vi "main.vi"() -> ()   [LabVIEW 2018]
panel:
  out "1#NG":bool
  out "外观NG":bool
  in  "选项卡控件":enum32{"外观检测", "左出风口"}(tab)
  out "1#海绵":bool
  out "3#小齿":bool
  out "3#海绵":bool
  out "3#缓冲块":bool
  out "3#内叶片":bool
  out "3#卡扣4":bool
  out "3#卡扣3":bool
  out "3#卡扣2":bool
  out "3#卡扣1":bool
  out "3#外观4":bool
  out "3#外观3":bool
  out "3#外观2":bool
  out "3#外观1":bool
  out "2#小齿":bool
  out "2#海绵":bool
  out "2#缓冲块":bool
  out "2#内叶片":bool
  out "2#卡扣4":bool
  out "2#卡扣3":bool
  out "2#卡扣2":bool
  out "2#卡扣1":bool
  out "2#外观4":bool
  out "2#外观3":bool
  out "2#外观2":bool
  out "2#外观1":bool
  out "1#小齿":bool
  out "1#缓冲块":bool
  out "1#内叶片":bool
  out "1#卡扣4":bool
  out "1#卡扣3":bool
  out "1#卡扣2":bool
  out "1#卡扣1":bool
  out "1#外观4":bool
  out "1#外观3":bool
  out "1#外观2":bool
  out "1#外观1":bool
  in  "外观检测结果":string
  out "图片1":picture
  out "图片4":picture
  out "图片3":picture
  out "图片2":picture
  out "1#F拨钮右左锁":string
  out "1#F拨钮右左":string
  out "1#F拨钮左右锁":string
  out "1#F拨钮左右":string
  out "1#拨钮左右标准":string
  out "1#拨钮左右锁止标准":string
  out "1#拨钮右左标准":string
  out "1#拨钮右左锁止标准":string
  out "1#泄漏量结果":string
  out "1#压力结果":string
  out "1#泄漏量标准":string
  in  "1#F选项卡控件":enum32{"拨钮左->右", "拨钮右->左", "拨钮下->上", "拨钮上->下"}(tab)
  out "1#拨钮左右":T1(graph) caption="拨钮左右"
  out "1#拨钮右左":T1(graph) caption="拨钮右左"
  out "1#拨钮下上":T2(graph) caption="拨钮下上"
  out "1#拨钮上下":T2(graph) caption="拨钮上下"
  out "1#压力标准":string
  out "1#拨钮下上标准":string
  out "1#拨钮上下标准":string
  out "1#F拨钮上下":string
  out "1#F拨钮下上":string
  out "产品名称":string="请选择出风口型号..."
  in  "产品选择":enum32{"未选择", "1", "2"}(radio)=enum."1"
  out "ROBOT通讯状态":bool
  out "PLC通讯":bool
  out "时刻":string
  in  "参数":bool
  in  "退出":bool
  out "OK-NG":string
  # "泄漏检测"
  # "拨钮操作力（N）"
  # "项目"
  # "标准"
  # "结果"
  # "操作方向"
  # "力类型"
  # "标准"
  # "结果"
  # "滑动力"
  # "上->下"
  # "压力"
  # "滑动力"
  # "下->上"
  # "泄漏量"
  # "拨钮操作力（N）"
  # "操作方向"
  # "力类型"
  # "标准"
  # "结果"
  # "滑动力"
  # "左->右"
  # "锁止力"
  # "滑动力"
  # "右->左"
  # "锁止力"
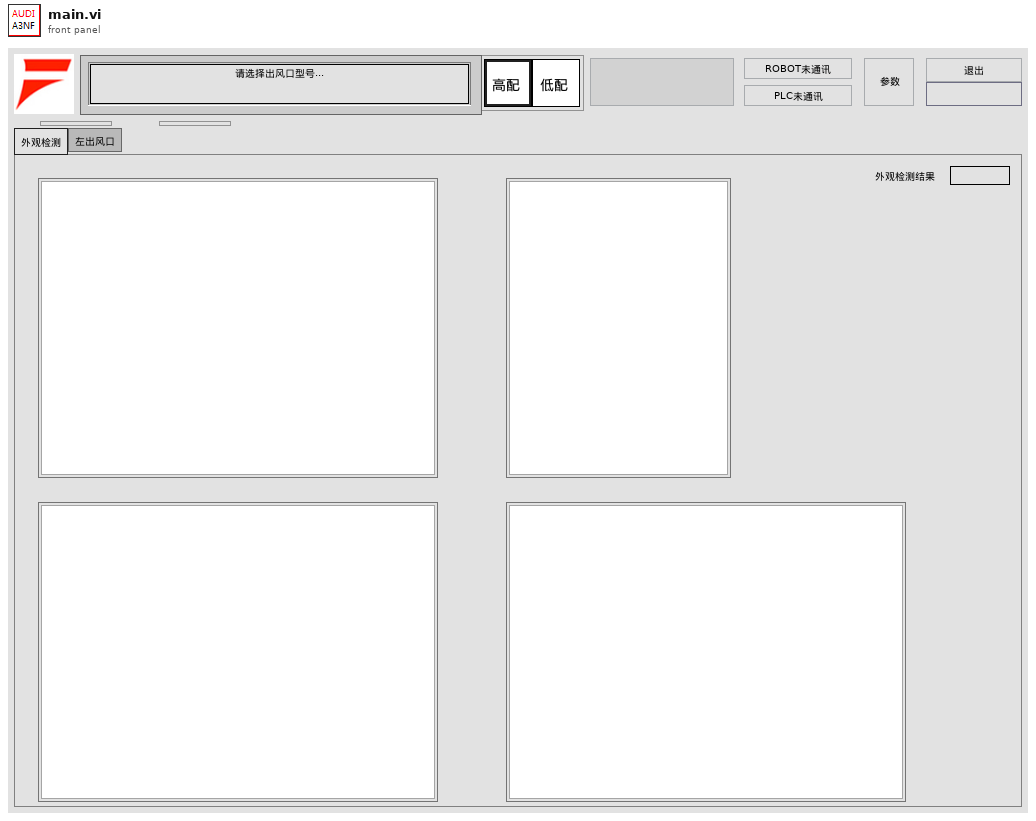
[diagram p1: front panel]
types:
  T1 = cluster{"力":sgl, "上限":sgl, "下限":sgl, "上参考":sgl, "下参考":sgl, "下参考 2":sgl}
  T2 = cluster{"力":sgl, "上限":sgl, "下限":sgl, "上参考":sgl, "下参考":sgl, "基准":sgl}
  T3 = enum8{"Enabled", "Disabled", "Disabled and Grayed Out"}
  T4 = cluster{"力":sgl, "上限":sgl, "下限":sgl, "上参考":sgl, "下参考":sgl, "下参考 2":sgl}[]
  T5 = enum32{"Invalid", "Standard", "Closed", "Hidden", "Minimized", "Maximized"}
  T6 = cluster{"压力":string, "泄漏量":string, "风门打开":string, "风门关闭":string, "LED电压":string, "LED电流":string, "拨钮左右":string, "拨钮左右锁止":string, "拨钮右左":string, "拨钮右左锁止":string, "拨钮上下":string, "拨钮下上":string, "轮盘关开":string, "轮盘关开锁止":string, "轮盘开关":string, "轮盘开关锁止":string}
  T7 = enum16{"Always On", "Always Off", "Off While Running"}
  T8 = cluster{"PLC就绪":bool, "ROBOT就绪":bool, "空动作":bool, "检测NG":bool, "检测结束":bool, "检测开始":bool, "初始化脉冲":bool, "1#检测NG":bool, "2#检测NG":bool, "3#检测NG":bool}
  T9 = cluster{"选择":enum16{"Fx", "Fy", "Fz", "Mx", "My", "Mz"}, "系数x":sgl, "系数+":sgl, "上限":sgl, "下限":sgl, "Ymax":dbl, "Ymin":dbl, "点数":dbl, "锁系数x":sgl, "锁上限":sgl, "锁下限":sgl, "锁系数+":sgl, "起点":dbl, "终点":dbl, "锁起点":dbl, "锁终点":dbl, "上参考":sgl, "下参考":sgl, "基准":sgl}
  T10 = cluster{"1#当前泄漏量":sgl, "1#稳定泄漏量":sgl, "1#当前压力":sgl, "1#稳定压力":sgl, "1#风门闭电压":sgl, "1#风门开电压":sgl, "1#LED电流":sgl, "1#LED电压":sgl, "2#当前泄漏量":sgl, "2#稳定泄漏量":sgl, "2#当前压力":sgl, "2#稳定压力":sgl, "2#风门闭电压":sgl, "2#风门开电压":sgl, "2#LED电流":sgl, "2#LED电压":sgl, "3#当前泄漏量":sgl, "3#稳定泄漏量":sgl, "3#当前压力":sgl, "3#稳定压力":sgl, "3#风门闭电压":sgl, "3#风门开电压":sgl, "3#LED电流":sgl, "3#LED电压":sgl}
  T11 = cluster{"泄漏量":bool, "风门开闭电检":bool, "LED电检":bool, "外观检测":bool, "1#轮盘关开":bool, "1#轮盘关开锁":bool, "1#轮盘开关":bool, "1#轮盘开关锁":bool, "1#拨钮左右":bool, "1#拨钮右左":bool, "1#拨钮上下":bool, "1#拨钮下上":bool, "2#轮盘关开":bool, "2#轮盘关开锁":bool, "2#轮盘开关":bool, "2#轮盘开关锁":bool, "2#拨钮左右":bool, "2#拨钮右左":bool, "2#拨钮上下":bool, "2#拨钮下上":bool, "3#轮盘关开":bool, "3#轮盘关开锁":bool, "3#轮盘开关":bool, "3#轮盘开关锁":bool, "3#拨钮左右":bool, "3#拨钮右左":bool, "3#拨钮上下":bool, "3#拨钮下上":bool}
  T12 = cluster{"1#泄漏量":bool, "1#风门闭电压":bool, "1#风门开电压":bool, "1#LED电压":bool, "1#LED电流":bool, "外观结果":bool, "2#泄漏量":bool, "2#风门闭电压":bool, "2#风门开电压":bool, "2#LED电压":bool, "2#LED电流":bool, "3#泄漏量":bool, "3#风门闭电压":bool, "3#风门开电压":bool, "3#LED电压":bool, "3#LED电流":bool}
  T13 = cluster{"主站IP":u32, "组号":u8, "帧号":u16, "时间戳":u64}
  T14 = cluster{"力":sgl, "上限":sgl, "下限":sgl, "上参考":sgl, "下参考":sgl, "基准":sgl}[]
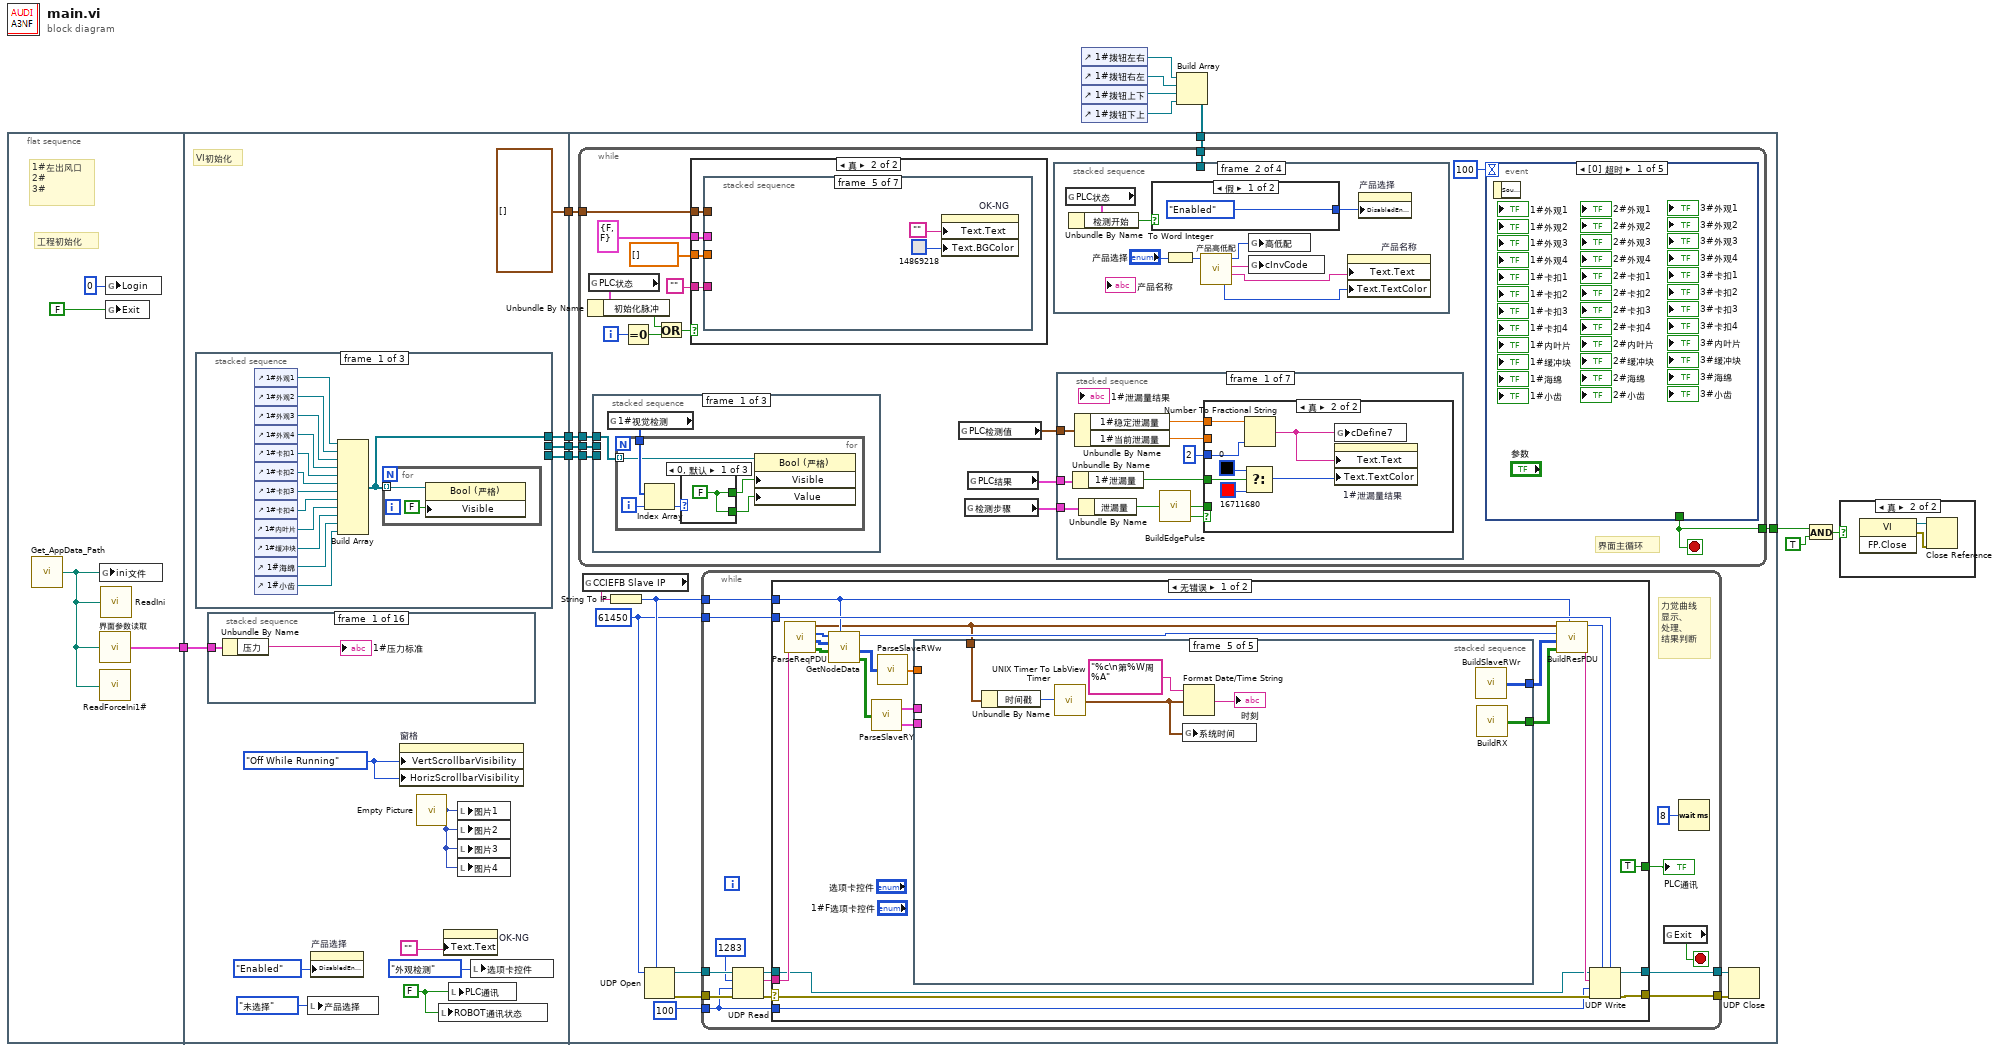
[diagram p0: block diagram]
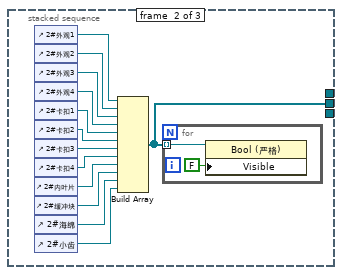
[diagram p2: hidden frame]
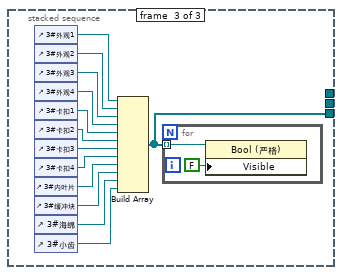
[diagram p3: hidden frame]
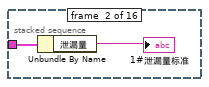
[diagram p4: hidden frame]
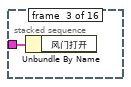
[diagram p5: hidden frame]
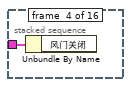
[diagram p6: hidden frame]
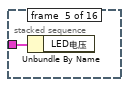
[diagram p7: hidden frame]
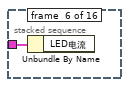
[diagram p8: hidden frame]
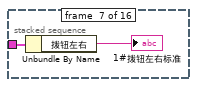
[diagram p9: hidden frame]
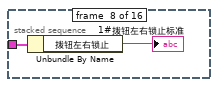
[diagram p10: hidden frame]
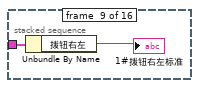
[diagram p11: hidden frame]
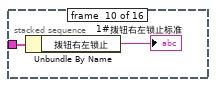
[diagram p12: hidden frame]
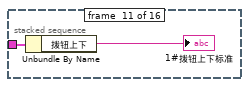
[diagram p13: hidden frame]
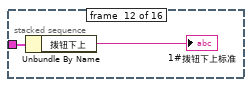
[diagram p14: hidden frame]
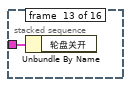
[diagram p15: hidden frame]
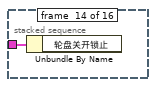
[diagram p16: hidden frame]
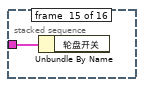
[diagram p17: hidden frame]
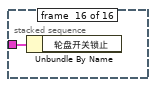
[diagram p18: hidden frame]
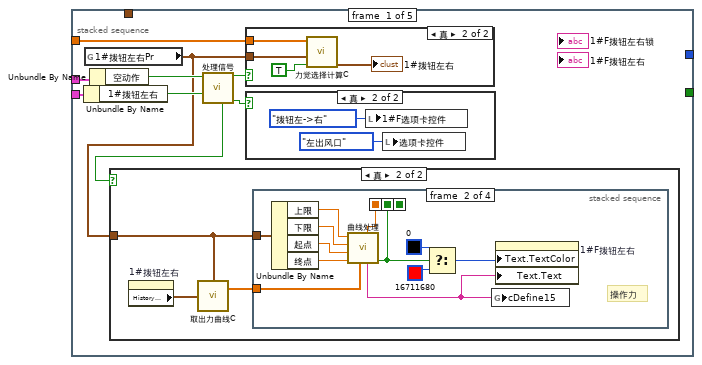
[diagram p19: hidden frame]
diagram:
  n1 = flat-sequence {
    tunnel: [w16] -> w9
    tunnel: [w29] -> w10
    tunnel: w9 -> [w26]
    tunnel: [w24] -> w8
    tunnel: [w23] -> w7
    tunnel: [T4 [] ("历史数据")] -> w6
    tunnel: [w112] -> w12
    tunnel: w10 -> [w105]
    tunnel: w8 -> [w102]
    tunnel: w7 -> [w101]
    tunnel: w6 -> [w100]
    tunnel: w1 -> [w99]
    frame #0 {
      # "1#左出风口\n2#\n3#"
      # "工程初始化"
      n2 = call "Get_AppData_Path.vi"() -> ("path"=w15:path)  [unwired: 1 in]
      n3 = global write "全局 1.vi" "ini文件"(w15) -> ()
      n4 = call "界面参数读取.vi"("路径"=w15) -> ("标准"=w16:T6)
      n5 = call "ReadForceIni1#.vi"("configuration file path"=w15) -> ()  [unwired: 1 in]
      n6 = call "ReadIni.vi"("configuration file path"=w15) -> ()  [unwired: 1 in]
      n7 = global write "全局 1.vi" "Login"(0 ("Login")) -> ()
      n8 = global write "全局 1.vi" "Exit"(FALSE ("退出")) -> ()
    }
    frame #1 {
      w25 = T7."Off While Running" ("垂直滚动条可见")
      w27 = FALSE
      # "VI初始化"
      n9 = stacked-sequence {
        tunnel: [w42 _ _] -> w29
        tunnel: [_ w45 _] -> w24
        tunnel: [_ _ w60] -> w23
        frame #0 {
          n10 = control-ref of="1#外观1"() -> (w30:refnum<vi>)
          n11 = control-ref of="1#外观2"() -> (w31:refnum<vi>)
          n12 = control-ref of="1#外观3"() -> (w32:refnum<vi>)
          n13 = control-ref of="1#外观4"() -> (w33:refnum<vi>)
          n14 = control-ref of="1#卡扣1"() -> (w34:refnum<vi>)
          n15 = control-ref of="1#卡扣2"() -> (w41:refnum<vi>)
          n16 = control-ref of="1#卡扣3"() -> (w40:refnum<vi>)
          n17 = control-ref of="1#卡扣4"() -> (w39:refnum<vi>)
          n18 = control-ref of="1#内叶片"() -> (w38:refnum<vi>)
          n19 = control-ref of="1#缓冲块"() -> (w37:refnum<vi>)
          n20 = control-ref of="1#海绵"() -> (w36:refnum<vi>)
          n21 = control-ref of="1#小齿"() -> (w35:refnum<vi>)
          n22 = Build Array(w30, w31, w32, w33, w34, w41, w40, w39, w38, w37, w36, w35) -> (w42:refnum<vi>[])
          n23 = for {
            tunnel: w42 -> [w43] mode=indexing
            n24 = property class="Bool (严格)"(reference=w43, "Visible"=FALSE ("可见")) -> ()  [unwired: 1 in, 2 out]
          }
        }
        frame #1 {
          n25 = control-ref of="2#外观1"() -> (w46:refnum<vi>)
          n26 = control-ref of="2#外观2"() -> (w47:refnum<vi>)
          n27 = control-ref of="2#外观3"() -> (w48:refnum<vi>)
          n28 = control-ref of="2#外观4"() -> (w49:refnum<vi>)
          n29 = control-ref of="2#卡扣1"() -> (w50:refnum<vi>)
          n30 = control-ref of="2#卡扣2"() -> (w57:refnum<vi>)
          n31 = control-ref of="2#卡扣3"() -> (w56:refnum<vi>)
          n32 = control-ref of="2#卡扣4"() -> (w55:refnum<vi>)
          n33 = control-ref of="2#内叶片"() -> (w54:refnum<vi>)
          n34 = control-ref of="2#缓冲块"() -> (w53:refnum<vi>)
          n35 = control-ref of="2#海绵"() -> (w52:refnum<vi>)
          n36 = control-ref of="2#小齿"() -> (w51:refnum<vi>)
          n37 = Build Array(w46, w47, w48, w49, w50, w57, w56, w55, w54, w53, w52, w51) -> (w45:refnum<vi>[])
          n38 = for {
            tunnel: w45 -> [w58] mode=indexing
            n39 = property class="Bool (严格)"(reference=w58, "Visible"=FALSE ("可见")) -> ()  [unwired: 1 in, 2 out]
          }
        }
        frame #2 {
          n40 = control-ref of="3#外观1"() -> (w61:refnum<vi>)
          n41 = control-ref of="3#外观2"() -> (w62:refnum<vi>)
          n42 = control-ref of="3#外观3"() -> (w63:refnum<vi>)
          n43 = control-ref of="3#外观4"() -> (w64:refnum<vi>)
          n44 = control-ref of="3#卡扣1"() -> (w65:refnum<vi>)
          n45 = control-ref of="3#卡扣2"() -> (w72:refnum<vi>)
          n46 = control-ref of="3#卡扣3"() -> (w71:refnum<vi>)
          n47 = control-ref of="3#卡扣4"() -> (w70:refnum<vi>)
          n48 = control-ref of="3#内叶片"() -> (w69:refnum<vi>)
          n49 = control-ref of="3#缓冲块"() -> (w68:refnum<vi>)
          n50 = control-ref of="3#海绵"() -> (w67:refnum<vi>)
          n51 = control-ref of="3#小齿"() -> (w66:refnum<vi>)
          n52 = Build Array(w61, w62, w63, w64, w65, w72, w71, w70, w69, w68, w67, w66) -> (w60:refnum<vi>[])
          n53 = for {
            tunnel: w60 -> [w73] mode=indexing
            n54 = property class="Bool (严格)"(reference=w73, "Visible"=FALSE ("可见")) -> ()  [unwired: 1 in, 2 out]
          }
        }
      }
      n55 = stacked-sequence {
        tunnel: w26 -> [w76 w78 w79 w80 w81 w82 w84 w86 w88 w90 w92 w94 w95 w96 w97 w98]
        frame #0 {
          n56 = Unbundle By Name(w76) -> ("压力"=→"1#压力标准":string)
        }
        frame #1 {
          n57 = Unbundle By Name(w78) -> ("泄漏量"=→"1#泄漏量标准":string)
        }
        frame #2 {
          n58 = Unbundle By Name(w79) -> ()  [unwired: 1 out]
        }
        frame #3 {
          n59 = Unbundle By Name(w80) -> ()  [unwired: 1 out]
        }
        frame #4 {
          n60 = Unbundle By Name(w81) -> ()  [unwired: 1 out]
        }
        frame #5 {
          n61 = Unbundle By Name(w82) -> ()  [unwired: 1 out]
        }
        frame #6 {
          n62 = Unbundle By Name(w84) -> ("拨钮左右"=→"1#拨钮左右标准":string)
        }
        frame #7 {
          n63 = Unbundle By Name(w86) -> ("拨钮左右锁止"=→"1#拨钮左右锁止标准":string)
        }
        frame #8 {
          n64 = Unbundle By Name(w88) -> ("拨钮右左"=→"1#拨钮右左标准":string)
        }
        frame #9 {
          n65 = Unbundle By Name(w90) -> ("拨钮右左锁止"=→"1#拨钮右左锁止标准":string)
        }
        frame #10 {
          n66 = Unbundle By Name(w92) -> ("拨钮上下"=→"1#拨钮上下标准":string)
        }
        frame #11 {
          n67 = Unbundle By Name(w94) -> ("拨钮下上"=→"1#拨钮下上标准":string)
        }
        frame #12 {
          n68 = Unbundle By Name(w95) -> ()  [unwired: 1 out]
        }
        frame #13 {
          n69 = Unbundle By Name(w96) -> ()  [unwired: 1 out]
        }
        frame #14 {
          n70 = Unbundle By Name(w97) -> ()  [unwired: 1 out]
        }
        frame #15 {
          n71 = Unbundle By Name(w98) -> ()  [unwired: 1 out]
        }
      }
      n72 = local write "产品选择"(enum32{"未选择", "1", "2"}."未选择" ("产品选择")) -> ()
      n73 = property on="产品选择" class="RadioBtnsControl (严格)"("DisabledEnum"=T3."Enabled" ("禁用")) -> ()  [unwired: 2 in, 2 out]
      n74 = property on="窗格" class="Pane"("VertScrollbarVisibility"=w25, "HorizScrollbarVisibility"=w25) -> ()  [unwired: 2 in, 2 out]
      n75 = call "Empty Picture"() -> ("empty picture"=w19:picture)
      n76 = local write "ROBOT通讯状态"(w27) -> ()
      n77 = property on="OK-NG" class="Str"("Text.Text"="") -> ()  [unwired: 2 in, 2 out]
      n78 = local write "PLC通讯"(w27) -> ()
      n79 = local write "图片1"(w19) -> ()
      n80 = local write "图片2"(w19) -> ()
      n81 = local write "图片3"(w19) -> ()
      n82 = local write "图片4"(w19) -> ()
      n83 = local write "选项卡控件"(enum32{"外观检测", "左出风口"}."外观检测" ("选项卡控件")) -> ()
    }
    frame #2 {
      w106 = u16 61450 ("端口")
      n84 = while {
        tunnel: [w362] -> w112
        tunnel: w105 -> [w361]
        tunnel: w102 -> [w354]
        tunnel: w101 -> [w353]
        tunnel: w100 -> [w347]
        tunnel: w99 -> [w346]
        i -> [w352]
        stop <- w362 stop-if-true
        # "界面主循环"
        n85 = global read "全局 1.vi" "PLC状态"() -> (w360:T8)
        n86 = Unbundle By Name(w360) -> ("初始化脉冲"=w350:bool)
        n87 = stacked-sequence {
          tunnel: w361 -> [w364 _ _]
          tunnel: w354 -> [_ w377 _]
          tunnel: w353 -> [_ _ w390]
          frame #0 {
            n88 = global read "全局 1.vi" "1#视觉检测"() -> (w365:u16[])
            n89 = for {
              tunnel: w364 -> [w366] mode=indexing
              tunnel: w365 -> [w371]
              i -> [w370]
              n90 = Index Array(array=w371, index=w370) -> (element=w369:u16)
              n91 = case shown="0, 默认" w369 {
                tunnel: [w372 TRUE TRUE] -> w368
                tunnel: [w372 FALSE TRUE] -> w367
                frame 0, Default {
                  w372 = FALSE
                }
                frame 1 {
                }
                frame 2 {
                }
              }
              n92 = property class="Bool (严格)"(reference=w366, "Visible"=w368, "Value"=w367) -> ()  [unwired: 1 in, 2 out]
            }
          }
          frame #1 {
            n93 = global read "全局 1.vi" "2#视觉检测"() -> (w378:u16[])
            n94 = for {
              tunnel: w377 -> [w379] mode=indexing
              tunnel: w378 -> [w384]
              i -> [w383]
              n95 = Index Array(array=w384, index=w383) -> (element=w382:u16)
              n96 = case shown="0, 默认" w382 {
                tunnel: [w385 TRUE TRUE] -> w381
                tunnel: [w385 FALSE TRUE] -> w380
                frame 0, Default {
                  w385 = FALSE
                }
                frame 1 {
                }
                frame 2 {
                }
              }
              n97 = property class="Bool (严格)"(reference=w379, "Visible"=w381, "Value"=w380) -> ()  [unwired: 1 in, 2 out]
            }
          }
          frame #2 {
            n98 = global read "全局 1.vi" "3#视觉检测"() -> (w391:u16[])
            n99 = for {
              tunnel: w390 -> [w392] mode=indexing
              tunnel: w391 -> [w397]
              i -> [w396]
              n100 = Index Array(array=w397, index=w396) -> (element=w395:u16)
              n101 = case shown="0, 默认" w395 {
                tunnel: [w398 TRUE TRUE] -> w394
                tunnel: [w398 FALSE TRUE] -> w393
                frame 0, Default {
                  w398 = FALSE
                }
                frame 1 {
                }
                frame 2 {
                }
              }
              n102 = property class="Bool (严格)"(reference=w392, "Visible"=w394, "Value"=w393) -> ()  [unwired: 1 in, 2 out]
            }
          }
        }
        n103 = Equal To 0?(x=w352) -> (x = 0?=w351:bool)
        n104 = Or(x=w350, y=w351) -> (x .or. y?=w349:bool)
        n105 = case shown="真" w349 {
          tunnel: cluster{bool, bool} {FALSE, FALSE} -> [_ w569]
          tunnel: sgl[] [] ("历史数据") -> [_ w568]
          tunnel: w347 -> [_ w567]
          tunnel: "" -> [_ w566]
          frame False {
          }
          frame True {
            n106 = stacked-sequence {
              tunnel: w569 -> [w578 w587 w596 w605 _ _ _]
              tunnel: w568 -> [_ _ _ _ _ _ _]
              tunnel: w567 -> [w570 w579 w589 w598 _ _ _]
              tunnel: w566 -> [w571 w580 w588 w597 _ w608 w610]
              frame #0 {
                n107 = global write "全局F结果.vi" "1#拨钮左右力检"(w578) -> ()
                n108 = global read "全局F参数.vi" "1#拨钮左右Pr"() -> (w576:T9)
                n109 = local write "1#F拨钮左右锁"(w571) -> ()
                n110 = local write "1#F拨钮左右"(w571) -> ()
                n111 = Unbundle By Name(w576) -> ("点数"=w577:dbl, "Ymax"=w573:dbl, "Ymin"=w572:dbl)
                n112 = Decrement(x=w577) -> (x-1=w575:dbl)
                n113 = property on="1#拨钮左右" class="WFChart (严格)"("History Data"=w570, "XScale.Minimum"=0.0, "XScale.Maximum"=w575, "YScale.Maximum"=w573, "YScale.Minimum"=w572) -> ()  [unwired: 2 in, 2 out]
              }
              frame #1 {
                n114 = global write "全局F结果.vi" "1#拨钮右左力检"(w587) -> ()
                n115 = global read "全局F参数.vi" "1#拨钮右左Pr"() -> (w586:T9)
                n116 = local write "1#F拨钮右左"(w580) -> ()
                n117 = local write "1#F拨钮右左锁"(w580) -> ()
                n118 = Unbundle By Name(w586) -> ("点数"=w585:dbl, "Ymax"=w584:dbl, "Ymin"=w583:dbl)
                n119 = Decrement(x=w585) -> (x-1=w582:dbl)
                n120 = property on="1#拨钮右左" class="WFChart (严格)"("History Data"=w579, "XScale.Minimum"=0.0 ("X标尺.范围:最大值"), "XScale.Maximum"=w582, "YScale.Maximum"=w584, "YScale.Minimum"=w583) -> ()  [unwired: 2 in, 2 out]
              }
              frame #2 {
                n121 = global read "全局F参数.vi" "1#拨钮下上Pr"() -> (w595:T9)
                n122 = global write "全局F结果.vi" "1#拨钮下上力检"(w596) -> ()
                n123 = local write "1#F拨钮下上"(w588) -> ()
                n124 = Unbundle By Name(w595) -> ("点数"=w594:dbl, "Ymax"=w591:dbl, "Ymin"=w590:dbl)
                n125 = Decrement(x=w594) -> (x-1=w593:dbl)
                n126 = property on="1#拨钮下上" class="WFChart (严格)"("History Data"=w589, "XScale.Minimum"=0.0 ("X标尺.范围:最大值"), "XScale.Maximum"=w593, "YScale.Maximum"=w591, "YScale.Minimum"=w590) -> ()  [unwired: 2 in, 2 out]
              }
              frame #3 {
                n127 = global write "全局F结果.vi" "1#拨钮上下力检"(w605) -> ()
                n128 = global read "全局F参数.vi" "1#拨钮上下Pr"() -> (w604:T9)
                n129 = local write "1#F拨钮上下"(w597) -> ()
                n130 = Unbundle By Name(w604) -> ("点数"=w603:dbl, "Ymax"=w600:dbl, "Ymin"=w599:dbl)
                n131 = Decrement(x=w603) -> (x-1=w602:dbl)
                n132 = property on="1#拨钮上下" class="WFChart (严格)"("History Data"=w598, "XScale.Minimum"=0.0 ("X标尺.范围:最大值"), "XScale.Maximum"=w602, "YScale.Maximum"=w600, "YScale.Minimum"=w599) -> ()  [unwired: 2 in, 2 out]
              }
              frame #4 {
                n133 = property on="OK-NG" class="Str"("Text.Text"="", "Text.BGColor"=u32 14869218) -> ()  [unwired: 2 in, 2 out]
              }
              frame #5 {
                n134 = local write "1#泄漏量结果"(w608) -> ()
                n135 = local write "1#压力结果"(w608) -> ()
              }
              frame #6 {
                w609 = FALSE
                n136 = local write "外观检测结果"(w610) -> ()
                n137 = local write "外观NG"(w609) -> ()
                n138 = local write "1#NG"(w609) -> ()
              }
            }
          }
        }
        n139 = global read "全局 1.vi" "PLC检测值"() -> (w358:T10)
        n140 = global read "全局 1.vi" "检测步骤"() -> (w359:T11)
        n141 = global read "全局 1.vi" "PLC结果"() -> (w357:T12)
        n142 = stacked-sequence {
          tunnel: w346 -> [_ _ _ w557]
          frame #0 {
            n143 = global read "全局 1.vi" "PLC状态"() -> (w531:T8)
            n144 = global read "全局 1.vi" "PC状态"() -> (w530:cluster{"PLC就绪":bool, "空动作中":bool})
            n145 = Bundle By Name(cluster=w530, "PLC就绪"=TRUE) -> (w528:cluster{"PLC就绪":bool, "空动作中":bool})
            n146 = Unbundle By Name(w531) -> ("ROBOT就绪"=→"ROBOT通讯状态":bool, "1#检测NG"=→"1#NG":bool)
            n147 = global write "全局 1.vi" "PC状态"(w528) -> ()
          }
          frame #1 {
            n148 = global read "全局 1.vi" "PLC状态"() -> (w541:T8)
            n149 = Unbundle By Name(w541) -> ("检测开始"=w540:bool)
            n150 = case shown="假" w540 {
              tunnel: [T3."Enabled" ("禁用") T3."Disabled and Grayed Out" ("禁用")] -> w539
              frame False {
              }
              frame True {
              }
            }
            n151 = To Word Integer(number="产品选择") -> (16bit integer=w537:i16)
            n152 = call "产品高低配.vi"("选择"=w537) -> ("颜色"=w534:u32, "产品名称"=w533:string, "物料编号"=w535:string, "高低配"=w536:i16)  [unwired: 5 in]
            n153 = global write "全局 1.vi" "高低配"(w536) -> ()
            n154 = global write "全局SQL.vi" "cInvCode"(w535) -> ()
            n155 = property on="产品名称" class="Str"("Text.Text"=w533, "Text.TextColor"=w534) -> ()  [unwired: 2 in, 2 out]
            n156 = property on="产品选择" class="RadioBtnsControl (严格)"("DisabledEnum"=w539) -> ()  [unwired: 2 in, 2 out]
          }
          frame #2 {
            n157 = global read "全局 1.vi" "PLC状态"() -> (w546:T8)
            n158 = Unbundle By Name(w546) -> ("检测NG"=w544:bool, "检测结束"=w545:bool)
            n159 = case shown="真" w545 {
              tunnel: w544 -> [_ w547]
              frame False {
              }
              frame True {
                n160 = case shown="假" w547 {
                  tunnel: ["合格" "不合格"] -> w550
                  tunnel: [u32 6618880 u32 16711680] -> w549
                  tunnel: [u32 0 u32 16448250] -> w548
                  frame False {
                  }
                  frame True {
                  }
                }
                n161 = property on="OK-NG" class="Str"("Text.Text"=w550, "Text.BGColor"=w549, "Text.TextColor"=w548) -> ()  [unwired: 2 in, 2 out]
              }
            }
          }
          frame #3 {
            n162 = global read "全局 1.vi" "PLC状态"() -> (w563:T8)
            n163 = Unbundle By Name(w563) -> ("检测NG"=w558:bool, "检测结束"=w559:bool)
            n164 = Compound Arithmetic op=AND ("复合运算")(w559, FALSE ("值")) -> (w562:bool)
            n165 = call "BuildEdgePulse.vi"("输入"=w562) -> ("下降沿"=w560:bool)  [unwired: 2 in, 2 out]
            n166 = case shown="真" w560 {
              tunnel: w558 -> [_ w565]
              tunnel: w557 -> [_ w564]
              frame False {
              }
              frame True {
                n167 = call "WriteDB.vi"("NG?"=w565, "曲线数组"=w564) -> ()  [unwired: 3 in]
              }
            }
          }
        }
        n168 = stacked-sequence {
          tunnel: w359 -> [w412 w436 w459 w474 w489 w503 w514]
          tunnel: w358 -> [w409 w433 w456 w471 w486 w500 _]
          tunnel: w357 -> [w405 w429 w453 w468 w483 w497 w511]
          frame #0 {
            n169 = Unbundle By Name(w405) -> ("1#泄漏量"=w404:bool)
            n170 = Unbundle By Name(w409) -> ("1#稳定泄漏量"=w407:sgl, "1#当前泄漏量"=w408:sgl)
            n171 = Unbundle By Name(w412) -> ("泄漏量"=w411:bool)
            n172 = call "BuildEdgePulse.vi"("输入"=w411) -> ("下降沿"=w410:bool, "输出"=w406:bool)  [unwired: 2 in, 1 out]
            n173 = case shown="真" w410 {
              tunnel: w408 -> [w415 _]
              tunnel: w407 -> [_ w426]
              tunnel: w406 -> [w414 _]
              tunnel: w404 -> [_ w425]
              tunnel: i16 2 ("精度(6)") -> [w413 w422]
              frame False {
                n174 = case shown="真" w414 {
                  tunnel: w415 -> [_ w419]
                  tunnel: w413 -> [_ w418]
                  frame False {
                  }
                  frame True {
                    n175 = Number To Fractional String(number=w419, precision (6)=w418) -> (F-format string=w416:string)  [unwired: 2 in]
                    n176 = property on="1#泄漏量结果" class="Str"("Text.Text"=w416, "Text.TextColor"=u32 0) -> ()  [unwired: 2 in, 2 out]
                  }
                }
              }
              frame True {
                n177 = Select(t=u32 0, s=w425, f=u32 16711680) -> (s? t:f=w421:u32)
                n178 = Number To Fractional String(number=w426, precision (6)=w422) -> (F-format string=w420:string)  [unwired: 2 in]
                n179 = global write "全局SQL.vi" "cDefine7"(w420) -> ()
                n180 = property on="1#泄漏量结果" class="Str"("Text.Text"=w420, "Text.TextColor"=w421) -> ()  [unwired: 2 in, 2 out]
              }
            }
          }
          frame #1 {
            n181 = Unbundle By Name(w429) -> ("1#泄漏量"=w428:bool)
            n182 = Unbundle By Name(w433) -> ("1#稳定压力"=w431:sgl, "1#当前压力"=w432:sgl)
            n183 = Unbundle By Name(w436) -> ("泄漏量"=w435:bool)
            n184 = call "BuildEdgePulse.vi"("输入"=w435) -> ("下降沿"=w434:bool, "输出"=w430:bool)  [unwired: 2 in, 1 out]
            n185 = case shown="假" w434 {
              tunnel: w432 -> [w439 _]
              tunnel: w431 -> [_ w449]
              tunnel: w430 -> [w438 _]
              tunnel: w428 -> [_ w448]
              tunnel: i16 1 ("精度(6)") -> [w437 w444]
              frame False {
                n186 = case shown="真" w438 {
                  tunnel: w439 -> [_ w441]
                  tunnel: w437 -> [_ w440]
                  frame False {
                  }
                  frame True {
                    n187 = Number To Fractional String(number=w441, precision (6)=w440) -> (F-format string=w443:string)  [unwired: 2 in]
                    n188 = property on="1#压力结果" class="Str"("Text.Text"=w443, "Text.TextColor"=u32 0) -> ()  [unwired: 2 in, 2 out]
                  }
                }
              }
              frame True {
                n189 = Select(t=u32 0, s=w448, f=u32 16711680) -> (s? t:f=w445:u32)
                n190 = Number To Fractional String(number=w449, precision (6)=w444) -> (F-format string=w450:string)  [unwired: 2 in]
                n191 = property on="1#压力结果" class="Str"("Text.Text"=w450, "Text.TextColor"=w445) -> ()  [unwired: 2 in, 2 out]
              }
            }
          }
          frame #2 {
            n192 = Unbundle By Name(w453) -> ("1#风门开电压"=w452:bool)
            n193 = Unbundle By Name(w459) -> ("风门开闭电检"=w458:bool)
            n194 = Unbundle By Name(w456) -> ("1#风门开电压"=w455:sgl)
            n195 = call "BuildEdgePulse.vi"("输入"=w458) -> ("下降沿"=w457:bool, "输出"=w454:bool)  [unwired: 2 in, 1 out]
            n196 = case shown="真" w457 {
              tunnel: w455 -> [_ w465]
              tunnel: w454 -> [_ _]
              tunnel: w452 -> [_ w464]
              tunnel: i16 2 ("精度(6)") -> [_ w461]
              frame False {
              }
              frame True {
                n197 = Number To Fractional String(number=w465, precision (6)=w461) -> (F-format string=w460:string)  [unwired: 2 in]
                n198 = Select(t=u32 0, s=w464, f=u32 16711680) -> ()  [unwired: 1 out]
                n199 = global write "全局SQL.vi" "cDefine17"(w460) -> ()
              }
            }
          }
          frame #3 {
            n200 = Unbundle By Name(w468) -> ("1#风门闭电压"=w467:bool)
            n201 = Unbundle By Name(w474) -> ("风门开闭电检"=w473:bool)
            n202 = Unbundle By Name(w471) -> ("1#风门闭电压"=w470:sgl)
            n203 = call "BuildEdgePulse.vi"("输入"=w473) -> ("下降沿"=w472:bool, "输出"=w469:bool)  [unwired: 2 in, 1 out]
            n204 = case shown="真" w472 {
              tunnel: w470 -> [_ w480]
              tunnel: w469 -> [_ _]
              tunnel: w467 -> [_ w479]
              tunnel: i16 2 ("精度(6)") -> [_ w476]
              frame False {
              }
              frame True {
                n205 = Number To Fractional String(number=w480, precision (6)=w476) -> (F-format string=w475:string)  [unwired: 2 in]
                n206 = Select(t=u32 0, s=w479, f=u32 16711680) -> ()  [unwired: 1 out]
                n207 = global write "全局SQL.vi" "cDefine18"(w475) -> ()
              }
            }
          }
          frame #4 {
            n208 = Unbundle By Name(w483) -> ("1#LED电压"=w482:bool)
            n209 = Unbundle By Name(w489) -> ("LED电检"=w488:bool)
            n210 = Unbundle By Name(w486) -> ("1#LED电压"=w485:sgl)
            n211 = call "BuildEdgePulse.vi"("输入"=w488) -> ("下降沿"=w487:bool, "输出"=w484:bool)  [unwired: 2 in, 1 out]
            n212 = case shown="真" w487 {
              tunnel: w485 -> [_ w494]
              tunnel: w484 -> [_ _]
              tunnel: w482 -> [_ w493]
              tunnel: i16 2 ("精度(6)") -> [_ w490]
              frame False {
              }
              frame True {
                n213 = Number To Fractional String(number=w494, precision (6)=w490) -> ()  [unwired: 2 in, 1 out]
                n214 = Select(t=u32 0, s=w493, f=u32 16711680) -> ()  [unwired: 1 out]
              }
            }
          }
          frame #5 {
            n215 = Unbundle By Name(w497) -> ("1#LED电流"=w496:bool)
            n216 = Unbundle By Name(w500) -> ("1#LED电流"=w499:sgl)
            n217 = Unbundle By Name(w503) -> ("LED电检"=w502:bool)
            n218 = call "BuildEdgePulse.vi"("输入"=w502) -> ("下降沿"=w501:bool, "输出"=w498:bool)  [unwired: 2 in, 1 out]
            n219 = case shown="真" w501 {
              tunnel: w499 -> [_ w509]
              tunnel: w498 -> [_ _]
              tunnel: w496 -> [_ w508]
              tunnel: i16 2 ("精度(6)") -> [_ w505]
              frame False {
              }
              frame True {
                n220 = Number To Fractional String(number=w509, precision (6)=w505) -> (F-format string=w504:string)  [unwired: 2 in]
                n221 = Select(t=u32 0, s=w508, f=u32 16711680) -> ()  [unwired: 1 out]
                n222 = global write "全局SQL.vi" "cDefine8"(w504) -> ()
              }
            }
          }
          frame #6 {
            n223 = Unbundle By Name(w514) -> ("外观检测"=w513:bool)
            n224 = Unbundle By Name(w511) -> ("外观结果"=w510:bool)
            n225 = call "BuildEdgePulse.vi"("输入"=w513) -> ("下降沿"=w512:bool, "上升沿"=w515:bool)  [unwired: 2 in, 1 out]
            n226 = case shown="真" w515 {
              frame False {
              }
              frame True {
                n227 = local write "选项卡控件"(enum32{"外观检测", "左出风口"}."外观检测" ("选项卡控件")) -> ()
              }
            }
            n228 = case shown="真" w512 {
              tunnel: w510 -> [_ w519]
              frame False {
              }
              frame True {
                n229 = case shown="真" w519 {
                  tunnel: ["NG" ("文本.文本") "OK" ("文本.文本")] -> w518
                  tunnel: [u32 16711680 u32 0] -> w517
                  tunnel: [TRUE FALSE] -> w516
                  frame False {
                  }
                  frame True {
                  }
                }
                "外观NG" <- w516
                n230 = property on="外观检测结果" class="Str"("Text.Text"=w518, "Text.TextColor"=w517) -> ()  [unwired: 2 in, 2 out]
              }
            }
          }
        }
        n231 = event shown="[0] 超时" {
          selector: _ -> [_ _ _ _ _]
          dyn-events: _ -> [_ _ _ _ _]
          timeout: 100 ("等待时间（毫秒）") -> [_ _ _ _ _]
          tunnel: [_ _ _ _ "退出"] -> w362
          event Timeout {
            n232 = event-data() -> ()  [unwired: 1 in, 1 out]
          }
          event "产品选择": Value Change {
            n233 = event-data() -> ("NewVal"=w615:enum32{"未选择", "1", "2"})  [unwired: 1 in]
            n234 = case shown="\"未选择\", 默认" w615 {
              tunnel: [w621 "G1.jpg" "D1.jpg"] -> w617
              tunnel: [w621 "G2.jpg" "D2.jpg"] -> w618
              tunnel: [w621 "G3.jpg" "D3.jpg"] -> w619
              frame "未选择", Default {
                w621 = ""
              }
              frame "1" {
              }
              frame "2" {
              }
            }
            n235 = global read "全局 1.vi" "ini文件"() -> (w620:path)
            n236 = call "显示JPEG图片.vi"("图片"=w617, "AppData路径"=w620) -> ("二维图片"=→"图片1":picture)
            n237 = call "显示JPEG图片.vi"("图片"=w618, "AppData路径"=w620) -> ("二维图片"=→"图片2":picture)
            n238 = call "显示JPEG图片.vi"("图片"=w619, "AppData路径"=w620) -> ("二维图片"=→"图片3":picture)
            n239 = call "显示JPEG图片.vi"("图片"="4.jpg", "AppData路径"=w620) -> ("二维图片"=→"图片4":picture)
          }
          event "参数": Mouse Up {
            w631 = FALSE ("结束前等待")
            n240 = event-data() -> ()  [unwired: 1 in, 1 out]
            n241 = vi-ref "参数.vi"() -> (w632:refnum<vi>)
            n242 = invoke class="VI" method="Run VI"(reference=w632, "Wait until done"=w631, "Auto Dispose Ref"=w631) -> (reference out=w630:refnum<vi>)  [unwired: 2 in, 4 out]
            n243 = invoke class="VI" method="FP.Open"(reference=w630) -> (reference out=w628:refnum<vi>, error out=w629:errorcluster)  [unwired: 4 in, 3 out]
            n244 = Close Reference(reference=w628, error in (no error)=w629) -> ()  [unwired: 1 out]
          }
          event "产品名称": Mouse Up {
            n245 = event-data() -> ()  [unwired: 1 in, 1 out]
            n246 = property class="VI"("FP.State"=T5."Minimized" ("前面板窗口:状态")) -> ()  [unwired: 2 in, 2 out]
          }
          event "退出": Value Change {
            n247 = event-data() -> ()  [unwired: 1 in, 1 out]
            n248 = global write "全局 1.vi" "Exit"("退出") -> ()
          }
        }
      }
      n249 = global read "全局 1.vi" "CCIEFB Slave IP"() -> (w104:string)
      n250 = String To IP(1:w104) -> (0:w107:u32)
      n251 = UDP Open(7:w107, 11:w106) -> (port=w111:refnum<k16>, 0:w109:errorcluster)  [unwired: 3 in, 1 out]
      n252 = while {
        tunnel: w111 -> [w126]
        tunnel: [w118] -> w110
        tunnel: w109 -> [w125]
        tunnel: [w116] -> w108
        tunnel: w107 -> [w120]
        tunnel: w106 -> [w119]
        tunnel: 100 ("超时毫秒(25000)") -> [w115]
        stop <- w114 stop-if-true
        # "力觉曲线\n显示、\n处理、\n结果判断"
        n253 = UDP Read(connection ID=w126, max size (548)=1283 ("最大值(548)"), timeout ms (25000)=w115, 8:w125) -> (data out=w123:string, error out=w124:errorcluster, 3:w121:refnum<k16>)  [unwired: 2 out]
        n254 = case shown="无错误" w124 {
          selector: w124 -> [w149 w342]
          tunnel: w123 -> [w145 _]
          tunnel: [w148 w341] -> w116
          tunnel: w121 -> [w127 w340]
          tunnel: w120 -> [w142 _]
          tunnel: w119 -> [w146 _]
          tunnel: [w147 w340] -> w118
          tunnel: w115 -> [w137 _]
          tunnel: [TRUE FALSE] -> w113
          frame No Error {
            n255 = call "ParseReqPDU.vi"("数据in"=w145) -> ("All RY"=w138:bool[][], "All RWw"=w139:u16[][], "从站IP组"=w141:u32[], "主站信息"=w128:T13)  [unwired: 7 in]
            n256 = call "GetNodeData.vi"("指定从站IP"=w142, "All RY in"=w138, "All RWw in"=w139, "从站IP组"=w141) -> ("Node RY"=w134:bool[][], "Node RWw"=w135:u16[][], "占用站数"=w140:i32)  [unwired: 5 in]
            n257 = call "ParseSlaveRY.vi"("RY"=w134) -> ("PLC状态"=w133:T8, "检测步骤"=w132:T11)
            n258 = call "ParseSlaveRWw.vi"("Node RWw"=w135) -> ("力觉力"=w136:sgl[])
            n259 = stacked-sequence {
              tunnel: w136 -> [w151 w202 w253 w293 _]
              tunnel: w133 -> [w158 w209 w260 w300 _]
              tunnel: w132 -> [w157 w208 w259 w299 _]
              tunnel: [_ _ _ _ w338] -> w131
              tunnel: [_ _ _ _ w337] -> w130
              tunnel: w128 -> [_ _ _ _ w336]
              frame #0 {
                n260 = Unbundle By Name(w157) -> ("1#拨钮左右"=w154:bool)
                n261 = global read "全局F参数.vi" "1#拨钮左右Pr"() -> (w150:T9)
                n262 = Unbundle By Name(w158) -> ("空动作"=w156:bool)
                n263 = call "处理信号.vi"("动作"=w154, "空动作"=w156) -> ("切换"=w155:bool, "显示曲线"=w153:bool, "判断"=w152:bool)  [unwired: 7 in]
                n264 = case shown="真" w152 {
                  tunnel: w150 -> [_ w167]
                  frame False {
                  }
                  frame True {
                    n265 = property on="1#拨钮左右" class="WFChart (严格)"() -> ("History Data"=w166:T4)  [unwired: 2 in, 2 out]
                    n266 = call "取出力曲线C.vi"("cPr"=w167, "历史数据"=w166) -> ("曲线"=w165:sgl[])  [unwired: 2 in, 1 out]
                    n267 = stacked-sequence {
                      seq-local: [_ w184 _ _] -> [_ _ _ w197]
                      seq-local: [_ w177 _ _] -> [_ _ w192 _]
                      seq-local: [_ _ w190 _] -> [_ _ _ w198]
                      tunnel: w167 -> [w168 w182 w189 _]
                      tunnel: w165 -> [w170 w183 w188 _]
                      frame #0 {
                        # "显示曲线"
                        n268 = call "捆绑力曲线C.vi"("力数组"=w170, "Pr"=w168) -> ("历史数据"=w169:T14)  [unwired: 1 in]
                        n269 = Array Size(array=w169) -> (size(s)=w173:i32)
                        n270 = Decrement(x=w173) -> (x-1=w172:i32)
                        n271 = To Double Precision Float(number=w172) -> (double precision float=w171:dbl)
                        n272 = property on="1#拨钮左右" class="WFChart (严格)"("History Data"=w169, "XScale.Maximum"=w171, "XScale.Minimum"=0.0 ("X标尺.范围:最小值")) -> ()  [unwired: 2 in, 2 out]
                      }
                      frame #1 {
                        # "操作力"
                        n273 = Unbundle By Name(w182) -> ("上限"=w181:sgl, "下限"=w180:sgl, "起点"=w179:dbl, "终点"=w178:dbl)
                        n274 = call "曲线处理.vi"("上限"=w181, "下限"=w180, "起点"=w179, "终点"=w178, "历史数据"=w183) -> ("值"=w177:sgl, "示值"=w175:string, "范围内?"=w184:bool)  [unwired: 2 in, 1 out]
                        n275 = Select(t=u32 0, s=w184, f=u32 16711680) -> (s? t:f=w185:u32)
                        n276 = global write "全局SQL.vi" "cDefine15"(w175) -> ()
                        n277 = property on="1#F拨钮左右" class="Str"("Text.TextColor"=w185, "Text.Text"=w175) -> ()  [unwired: 2 in, 2 out]
                      }
                      frame #2 {
                        # "锁止力"
                        n278 = call "曲线处理C.vi"("基值"=w192, "历史数据"=w188, "Pr"=w189) -> ("范围内?"=w190:bool, "示值+"=w187:string)  [unwired: 5 in, 2 out]
                        n279 = Select(t=u32 0, s=w190, f=u32 16711680) -> (s? t:f=w193:u32)
                        n280 = property on="1#F拨钮左右锁" class="Str"("Text.TextColor"=w193, "Text.Text"=w187) -> ()  [unwired: 2 in, 2 out]
                        n281 = global write "全局SQL.vi" "cDefine16"(w187) -> ()
                      }
                      frame #3 {
                        n282 = Not And(1:w197, 2:w198) -> (0:w199:bool)
                        n283 = Bundle By Name(cluster=cluster{"判断完成":bool, "不合格?":bool} {"判断完成"=FALSE, "不合格?"=FALSE} ("1#轮盘关开力检"), "判断完成"=TRUE, "不合格?"=w199) -> (w195:cluster{"判断完成":bool, "不合格?":bool})
                        n284 = global write "全局F结果.vi" "1#拨钮左右力检"(w195) -> ()
                      }
                    }
                  }
                }
                n285 = case shown="真" w153 {
                  tunnel: w151 -> [_ w164]
                  tunnel: w150 -> [_ w163]
                  frame False {
                  }
                  frame True {
                    n286 = call "力觉选择计算C.vi"("取绝对值?F"=TRUE, "Pr"=w163, "力"=w164) -> ("六曲线"=→"1#拨钮左右":T2)  [unwired: 7 in, 1 out]
                  }
                }
                n287 = case shown="真" w155 {
                  frame False {
                  }
                  frame True {
                    n288 = local write "1#F选项卡控件"(enum32{"拨钮左->右", "拨钮右->左", "拨钮下->上", "拨钮上->下"}."拨钮左->右" ("1#F选项卡控件")) -> ()
                    n289 = local write "选项卡控件"(enum32{"外观检测", "左出风口"}."左出风口" ("选项卡控件")) -> ()
                  }
                }
              }
              frame #1 {
                n290 = global read "全局F参数.vi" "1#拨钮右左Pr"() -> (w201:T9)
                n291 = Unbundle By Name(w208) -> ("1#拨钮右左"=w204:bool)
                n292 = Unbundle By Name(w209) -> ("空动作"=w207:bool)
                n293 = call "处理信号.vi"("动作"=w204, "空动作"=w207) -> ("切换"=w205:bool, "显示曲线"=w206:bool, "判断"=w203:bool)  [unwired: 7 in]
                n294 = case shown="真" w203 {
                  tunnel: w201 -> [_ w217]
                  frame False {
                  }
                  frame True {
                    n295 = property on="1#拨钮右左" class="WFChart (严格)"() -> ("History Data"=w218:T4)  [unwired: 2 in, 2 out]
                    n296 = call "取出力曲线C.vi"("cPr"=w217, "历史数据"=w218) -> ("曲线"=w216:sgl[])  [unwired: 2 in, 1 out]
                    n297 = stacked-sequence {
                      seq-local: [_ w234 _ _] -> [_ _ _ w247]
                      seq-local: [_ w229 _ _] -> [_ _ w243 _]
                      seq-local: [_ _ w241 _] -> [_ _ _ w248]
                      tunnel: w217 -> [w219 w232 w240 _]
                      tunnel: w216 -> [w221 w233 w239 _]
                      frame #0 {
                        # "显示曲线"
                        n298 = call "捆绑力曲线C.vi"("力数组"=w221, "Pr"=w219) -> ("历史数据"=w220:T14)  [unwired: 1 in]
                        n299 = Array Size(array=w220) -> (size(s)=w224:i32)
                        n300 = Decrement(x=w224) -> (x-1=w223:i32)
                        n301 = To Double Precision Float(number=w223) -> (double precision float=w222:dbl)
                        n302 = property on="1#拨钮右左" class="WFChart (严格)"("History Data"=w220, "XScale.Maximum"=w222, "XScale.Minimum"=0.0 ("X标尺.范围:最小值")) -> ()  [unwired: 2 in, 2 out]
                      }
                      frame #1 {
                        # "操作力"
                        n303 = Unbundle By Name(w232) -> ("上限"=w231:sgl, "下限"=w230:sgl, "起点"=w228:dbl, "终点"=w227:dbl)
                        n304 = call "曲线处理.vi"("上限"=w231, "下限"=w230, "起点"=w228, "终点"=w227, "历史数据"=w233) -> ("值"=w229:sgl, "示值"=w226:string, "范围内?"=w234:bool)  [unwired: 2 in, 1 out]
                        n305 = Select(t=u32 0, s=w234, f=u32 16711680) -> (s? t:f=w235:u32)
                        n306 = global write "全局SQL.vi" "cDefine11"(w226) -> ()
                        n307 = property on="1#F拨钮右左" class="Str"("Text.TextColor"=w235, "Text.Text"=w226) -> ()  [unwired: 2 in, 2 out]
                      }
                      frame #2 {
                        # "锁止力"
                        n308 = call "曲线处理C.vi"("基值"=w243, "历史数据"=w239, "Pr"=w240) -> ("范围内?"=w241:bool, "示值+"=w238:string)  [unwired: 5 in, 2 out]
                        n309 = Select(t=u32 0, s=w241, f=u32 16711680) -> (s? t:f=w244:u32)
                        n310 = property on="1#F拨钮右左锁" class="Str"("Text.TextColor"=w244, "Text.Text"=w238) -> ()  [unwired: 2 in, 2 out]
                        n311 = global write "全局SQL.vi" "cDefine12"(w238) -> ()
                      }
                      frame #3 {
                        n312 = Not And(1:w247, 2:w248) -> (0:w249:bool)
                        n313 = Bundle By Name(cluster=cluster{"判断完成":bool, "不合格?":bool} {"判断完成"=FALSE, "不合格?"=FALSE} ("1#轮盘开关力检"), "判断完成"=TRUE, "不合格?"=w249) -> (w251:cluster{"判断完成":bool, "不合格?":bool})
                        n314 = global write "全局F结果.vi" "1#拨钮右左力检"(w251) -> ()
                      }
                    }
                  }
                }
                n315 = case shown="真" w205 {
                  frame False {
                  }
                  frame True {
                    n316 = local write "1#F选项卡控件"(enum32{"拨钮左->右", "拨钮右->左", "拨钮下->上", "拨钮上->下"}."拨钮右->左" ("1#F选项卡控件")) -> ()
                    n317 = local write "选项卡控件"(enum32{"外观检测", "左出风口"}."左出风口" ("选项卡控件")) -> ()
                  }
                }
                n318 = case shown="真" w206 {
                  tunnel: w202 -> [_ w215]
                  tunnel: w201 -> [_ w214]
                  frame False {
                  }
                  frame True {
                    n319 = call "力觉选择计算C.vi"("取绝对值?F"=TRUE, "Pr"=w214, "力"=w215) -> ("六曲线"=→"1#拨钮右左":T2)  [unwired: 7 in, 1 out]
                  }
                }
              }
              frame #2 {
                n320 = Unbundle By Name(w259) -> ("1#拨钮上下"=w254:bool)
                n321 = global read "全局F参数.vi" "1#拨钮上下Pr"() -> (w252:T9)
                n322 = Unbundle By Name(w260) -> ("空动作"=w257:bool)
                n323 = call "处理信号.vi"("动作"=w254, "空动作"=w257) -> ("切换"=w256:bool, "显示曲线"=w255:bool, "判断"=w258:bool)  [unwired: 7 in]
                n324 = case shown="真" w258 {
                  tunnel: w252 -> [_ w262]
                  frame False {
                  }
                  frame True {
                    n325 = property on="1#拨钮上下" class="WFChart (严格)"() -> ("History Data"=w263:T14)  [unwired: 2 in, 2 out]
                    n326 = call "取出力曲线C.vi"("cPr"=w262, "截取?F"=TRUE, "历史数据"=w263) -> ("曲线"=w261:sgl[])  [unwired: 1 in, 1 out]
                    n327 = stacked-sequence {
                      seq-local: [_ w274 _] -> [_ _ w282]
                      tunnel: w261 -> [w271 w280 _]
                      tunnel: w262 -> [w265 w272 _]
                      frame #0 {
                        n328 = call "捆绑力曲线C.vi"("力数组"=w271, "Pr"=w265) -> ("历史数据"=w266:T14)  [unwired: 1 in]
                        n329 = Array Size(array=w266) -> (size(s)=w270:i32)
                        n330 = To Double Precision Float(number=w270) -> (double precision float=w269:dbl)
                        n331 = Decrement(x=w269) -> (x-1=w268:dbl)
                        n332 = property on="1#拨钮上下" class="WFChart (严格)"("History Data"=w266, "XScale.Maximum"=w268, "XScale.Minimum"=0.0 ("X标尺.范围:最小值")) -> ()  [unwired: 2 in, 2 out]
                      }
                      frame #1 {
                        n333 = Unbundle By Name(w272) -> ("上限"=w279:sgl, "下限"=w278:sgl)
                        n334 = call "曲线处理.vi"("上限"=w279, "下限"=w278, "历史数据"=w280) -> ("示值"=w273:string, "范围内?"=w274:bool)  [unwired: 4 in, 2 out]
                        n335 = Select(t=u32 0, s=w274, f=u32 16711680) -> (s? t:f=w277:u32)
                        n336 = property on="1#F拨钮上下" class="Str"("Text.TextColor"=w277, "Text.Text"=w273) -> ()  [unwired: 2 in, 2 out]
                        n337 = global write "全局SQL.vi" "cDefine9"(w273) -> ()
                      }
                      frame #2 {
                        n338 = Not(x=w282) -> (.not. x?=w285:bool)
                        n339 = Bundle By Name(cluster=cluster{"判断完成":bool, "不合格?":bool} {"判断完成"=FALSE, "不合格?"=FALSE} ("1#拨钮上下力检"), "判断完成"=TRUE, "不合格?"=w285) -> (w284:cluster{"判断完成":bool, "不合格?":bool})
                        n340 = global write "全局F结果.vi" "1#拨钮上下力检"(w284) -> ()
                      }
                    }
                  }
                }
                n341 = case shown="真" w255 {
                  tunnel: w253 -> [_ w291]
                  tunnel: w252 -> [_ w290]
                  frame False {
                  }
                  frame True {
                    n342 = call "力觉选择计算C.vi"("取绝对值?F"=TRUE, "Pr"=w290, "力"=w291) -> ("六曲线"=→"1#拨钮上下":T2)  [unwired: 7 in, 1 out]
                  }
                }
                n343 = case shown="真" w256 {
                  frame False {
                  }
                  frame True {
                    n344 = local write "1#F选项卡控件"(enum32{"拨钮左->右", "拨钮右->左", "拨钮下->上", "拨钮上->下"}."拨钮上->下" ("1#F选项卡控件")) -> ()
                    n345 = local write "选项卡控件"(enum32{"外观检测", "左出风口"}."左出风口" ("选项卡控件")) -> ()
                  }
                }
              }
              frame #3 {
                n346 = global read "全局F参数.vi" "1#拨钮下上Pr"() -> (w292:T9)
                n347 = Unbundle By Name(w299) -> ("1#拨钮下上"=w294:bool)
                n348 = Unbundle By Name(w300) -> ("空动作"=w298:bool)
                n349 = call "处理信号.vi"("动作"=w294, "空动作"=w298) -> ("切换"=w296:bool, "显示曲线"=w297:bool, "判断"=w295:bool)  [unwired: 7 in]
                n350 = case shown="真" w295 {
                  tunnel: w292 -> [_ w302]
                  frame False {
                  }
                  frame True {
                    n351 = property on="1#拨钮下上" class="WFChart (严格)"() -> ("History Data"=w304:T14)  [unwired: 2 in, 2 out]
                    n352 = call "取出力曲线C.vi"("cPr"=w302, "截取?F"=TRUE, "历史数据"=w304) -> ("曲线"=w301:sgl[])  [unwired: 1 in, 1 out]
                    n353 = stacked-sequence {
                      seq-local: [_ w314 _] -> [_ _ w322]
                      tunnel: w301 -> [w311 w320 _]
                      tunnel: w302 -> [w305 w312 _]
                      frame #0 {
                        n354 = call "捆绑力曲线C.vi"("力数组"=w311, "Pr"=w305) -> ("历史数据"=w306:T14)  [unwired: 1 in]
                        n355 = Array Size(array=w306) -> (size(s)=w310:i32)
                        n356 = To Double Precision Float(number=w310) -> (double precision float=w309:dbl)
                        n357 = Decrement(x=w309) -> (x-1=w308:dbl)
                        n358 = property on="1#拨钮下上" class="WFChart (严格)"("History Data"=w306, "XScale.Maximum"=w308, "XScale.Minimum"=0.0 ("X标尺.范围:最小值")) -> ()  [unwired: 2 in, 2 out]
                      }
                      frame #1 {
                        n359 = Unbundle By Name(w312) -> ("上限"=w319:sgl, "下限"=w318:sgl)
                        n360 = call "曲线处理.vi"("上限"=w319, "下限"=w318, "历史数据"=w320) -> ("示值"=w313:string, "范围内?"=w314:bool)  [unwired: 4 in, 2 out]
                        n361 = Select(t=u32 0, s=w314, f=u32 16711680) -> (s? t:f=w317:u32)
                        n362 = global write "全局SQL.vi" "cDefine13"(w313) -> ()
                        n363 = property on="1#F拨钮下上" class="Str"("Text.TextColor"=w317, "Text.Text"=w313) -> ()  [unwired: 2 in, 2 out]
                      }
                      frame #2 {
                        n364 = Not(x=w322) -> (.not. x?=w325:bool)
                        n365 = Bundle By Name(cluster=cluster{"判断完成":bool, "不合格?":bool} {"判断完成"=FALSE, "不合格?"=FALSE} ("1#拨钮下上力检"), "判断完成"=TRUE, "不合格?"=w325) -> (w324:cluster{"判断完成":bool, "不合格?":bool})
                        n366 = global write "全局F结果.vi" "1#拨钮下上力检"(w324) -> ()
                      }
                    }
                  }
                }
                n367 = case shown="真" w297 {
                  tunnel: w293 -> [_ w331]
                  tunnel: w292 -> [_ w330]
                  frame False {
                  }
                  frame True {
                    n368 = call "力觉选择计算C.vi"("取绝对值?F"=TRUE, "Pr"=w330, "力"=w331) -> ("六曲线"=→"1#拨钮下上":T2)  [unwired: 7 in, 1 out]
                  }
                }
                n369 = case shown="真" w296 {
                  frame False {
                  }
                  frame True {
                    n370 = local write "1#F选项卡控件"(enum32{"拨钮左->右", "拨钮右->左", "拨钮下->上", "拨钮上->下"}."拨钮下->上" ("1#F选项卡控件")) -> ()
                    n371 = local write "选项卡控件"(enum32{"外观检测", "左出风口"}."左出风口" ("选项卡控件")) -> ()
                  }
                }
              }
              frame #4 {
                n372 = Unbundle By Name(w336) -> ("时间戳"=w335:u64)
                n373 = call "UNIX Timer To LabView Timer.vi"("UNIX时间戳"=w335) -> ("LabVIEW时间标识"=w332:timestamp)
                n374 = global write "全局 1.vi" "系统时间"(w332) -> ()
                n375 = Format Date/Time String(time format string (%c)="%c\n第%W周 %A" ("时间格式字符串(%c)"), seconds (now)=w332) -> (date/time string=→"时刻":string)  [unwired: 1 in]
                n376 = call "BuildSlaveRWr.vi"() -> ("RWr"=w337:i16[][])  [unwired: 1 in]
                n377 = call "BuildRX.vi"() -> ("RX"=w338:bool[][])  [unwired: 6 in]
              }
            }
            n378 = call "BuildResPDU.vi"("从站IP"=w142, "Node RX"=w131, "Node RWr"=w130, "占用站数"=w140, "主站信息"=w128) -> ("输出字符串"=w144:string, "主站IP"=w143:u32)  [unwired: 5 in]
            n379 = UDP Write(address=w143, port or service name=w146, connection ID=w127, data in=w144, 8:w149, 9:w137) -> (error out=w148:errorcluster, 3:w147:refnum<k16>)
          }
          frame Error {
            n380 = Unbundle By Name(w342) -> ("code"=w343:i32)
            n381 = case shown="56" w343 {
              tunnel: [w344 w345] -> w341
              tunnel: w342 -> [w344 _]
              frame Default {
              }
              frame 56 {
                w345 = errorcluster {"status"=FALSE, "code"=0, "source"=""}  # 无错误
              }
            }
          }
        }
        "PLC通讯" <- w113
        n382 = global read "全局 1.vi" "Exit"() -> (w114:bool)
        n383 = Wait (ms)(milliseconds to wait=u32 8 ("等待时间（毫秒）")) -> ()  [unwired: 1 out]
      }
      n384 = UDP Close(connection ID=w110, 8:w108) -> ()  [unwired: 2 out]
    }
  }
  n385 = control-ref of="1#拨钮左右"() -> (w5:refnum<vi>)
  n386 = control-ref of="1#拨钮右左"() -> (w4:refnum<vi>)
  n387 = control-ref of="1#拨钮上下"() -> (w3:refnum<vi>)
  n388 = control-ref of="1#拨钮下上"() -> (w2:refnum<vi>)
  n389 = Build Array(w5, w4, w3, w2) -> (w1:refnum<vi>[])
  n390 = And(x=w12, y=TRUE) -> (x .and. y?=w11:bool)
  n391 = case shown="真" w11 {
    frame False {
    }
    frame True {
      n392 = invoke class="VI" method="FP.Close"() -> (reference out=w635:refnum<vi>, error out=w636:errorcluster)  [unwired: 3 in, 1 out]
      n393 = Close Reference(reference=w635, error in (no error)=w636) -> ()  [unwired: 1 out]
    }
  }
